vi "API Set Run.vi"(8 "error in":errorcluster, 10 "Air Temperature Setpoint":dbl min=-200.0 max=300.0 step=1.0 format="%.1f", 11 "VISA resource name":refnum<visa-resource-name>) -> (0 "error out":errorcluster, 3 "VISA resource name out":refnum<visa-resource-name>)   [LabVIEW 2024, in "Thermotron 8800.lvlib"]
uses:
  Thermotron 8800.lvlib
  Private/get set.ctl
  Private/AnalogInputChannelNumber 1-4.ctl
  97e2181b-2865-4989-9e4d-9a6dd287fb6f.vi
  3f190baf-6335-4004-9e79-387b8d9bfee6.vi
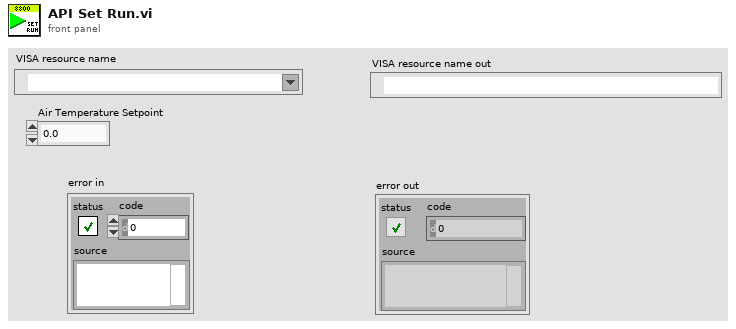
[diagram p1: front panel]
types:
  T1 = typedef "Thermotron 8800.lvlib/AnalogInputChannelNumber 1-4.ctl" = u16
  T2 = typedef "Thermotron 8800.lvlib/get set.ctl" = enum16{"get", "set"}
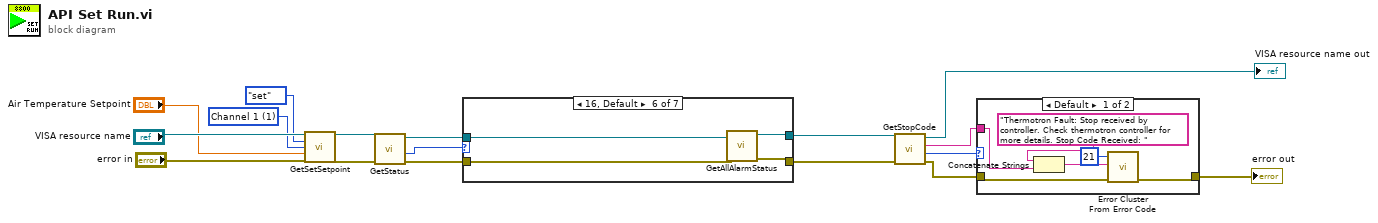
[diagram p0: block diagram]
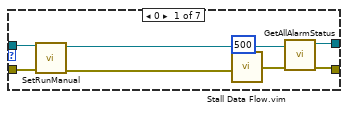
[diagram p3: hidden frame]
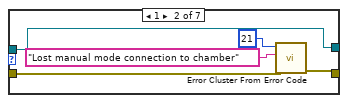
[diagram p4: hidden frame]
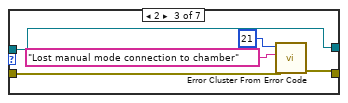
[diagram p5: hidden frame]
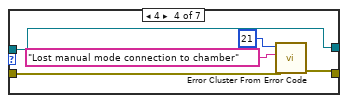
[diagram p6: hidden frame]
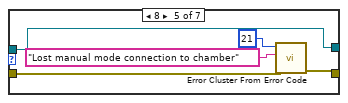
[diagram p7: hidden frame]
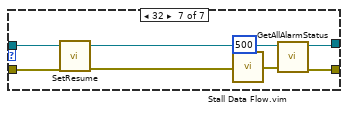
[diagram p8: hidden frame]
diagram:
  w2 = T1 1 items=["Channel 1"=1, "Channel 2"=2, "Channel 3"=3, "Channel 4"=4] ("Channel Number (1-4)")
  n1 = call "GetSetSetpoint.vi"("VISA resource name"="VISA resource name", "get/set"=get_set."set", "Channel Number (1-4)"=w2, "Setpoint"="Air Temperature Setpoint", "error in"="error in") -> ("VISA resource name out"=w7:refnum<visa-resource-name>, "error out"=w6:errorcluster)  [unwired: 7 in, 2 out]
  n2 = call "GetStatus.vi"("error in"=w6, "VISA resource name"=w7) -> ("error out"=w15:errorcluster, "Status word"=w17:i32, "VISA resource name out"=w16:refnum<visa-resource-name>)  [unwired: 6 in, 1 out]
  n3 = case shown="16, Default" w17 {
    tunnel: [w20 w27 w32 w37 w42 w48 w54] -> w13
    tunnel: w15 -> [w24 w28 w33 w38 w43 w46 w55]
    tunnel: w16 -> [w23 w26 w31 w36 w41 w47 w56]
    tunnel: [w21 w26 w31 w36 w41 w49 w53] -> w14
    frame 0 {
      n4 = call "SetRunManual.vi"("error in"=w24, "VISA resource name"=w23) -> ("error out"=w22:errorcluster, "VISA resource name out"=w18:refnum<visa-resource-name>)  [unwired: 7 in, 1 out]
      n5 = call "Stall Data Flow.vim"("value in"=w22, "milliseconds to wait"=u32 500) -> ("value out"=w19:errorcluster)  [unwired: 1 out]
      n6 = call "GetAllAlarmStatus.vi"("error in"=w19, "VISA resource name"=w18) -> ("error out"=w20:errorcluster, "VISA resource name out"=w21:refnum<visa-resource-name>)  [unwired: 8 in]
    }
    frame 1 {
      n7 = call <vilib>:"Error Cluster From Error Code.vi"("error in (no error)"=w28, "error message (\"\")"="Lost manual mode connection to chamber" ("error message (\"\")"), "error code (0)"=21) -> ("error out"=w27:errorcluster)  [unwired: 6 in]
    }
    frame 2 {
      n8 = call <vilib>:"Error Cluster From Error Code.vi"("error in (no error)"=w33, "error message (\"\")"="Lost manual mode connection to chamber" ("error message (\"\")"), "error code (0)"=21) -> ("error out"=w32:errorcluster)  [unwired: 6 in]
    }
    frame 4 {
      n9 = call <vilib>:"Error Cluster From Error Code.vi"("error in (no error)"=w38, "error message (\"\")"="Lost manual mode connection to chamber" ("error message (\"\")"), "error code (0)"=21) -> ("error out"=w37:errorcluster)  [unwired: 6 in]
    }
    frame 8 {
      n10 = call <vilib>:"Error Cluster From Error Code.vi"("error in (no error)"=w43, "error message (\"\")"="Lost manual mode connection to chamber" ("error message (\"\")"), "error code (0)"=21) -> ("error out"=w42:errorcluster)  [unwired: 6 in]
    }
    frame 16, Default {
      n11 = call "GetAllAlarmStatus.vi"("error in"=w46, "VISA resource name"=w47) -> ("error out"=w48:errorcluster, "VISA resource name out"=w49:refnum<visa-resource-name>)  [unwired: 8 in]
    }
    frame 32 {
      n12 = call "SetResume.vi"("error in"=w55, "VISA resource name"=w56) -> ("error out"=w50:errorcluster, "VISA resource name out"=w51:refnum<visa-resource-name>)  [unwired: 7 in, 1 out]
      n13 = call "Stall Data Flow.vim"("value in"=w50, "milliseconds to wait"=u32 500) -> ("value out"=w52:errorcluster)  [unwired: 1 out]
      n14 = call "GetAllAlarmStatus.vi"("error in"=w52, "VISA resource name"=w51) -> ("error out"=w54:errorcluster, "VISA resource name out"=w53:refnum<visa-resource-name>)  [unwired: 8 in]
    }
  }
  n15 = call "GetStopCode.vi"("error in"=w13, "VISA resource name"=w14) -> ("error out"=w12:errorcluster, 1:"Stop code"=w10:i32, 2:"Stop code"=w11:string, "VISA resource name out"=→"VISA resource name out":refnum<visa-resource-name>)  [unwired: 6 in]
  n16 = case shown="Default" w10 {
    tunnel: w12 -> [w63 w64]
    tunnel: [w62 w64] -> w8
    tunnel: w11 -> [w58 _]
    frame Default {
      n17 = Concatenate Strings("Thermotron Fault: Stop received by controller. Check thermotron controller for more details. Stop Code Received: " ("error message (\"\")"), w58) -> (w59:string)
      n18 = call <vilib>:"Error Cluster From Error Code.vi"("error in (no error)"=w63, "error message (\"\")"=w59, "error code (0)"=21) -> ("error out"=w62:errorcluster)  [unwired: 6 in]
    }
    frame 0, 1 {
    }
  }
  "error out" <- w8
